vi "Dark Array FGV.vi"(10 "Control":enum16{"get", "add", "reset"}(ring), 11 "Next Dark Measurement In":dbl[][](array[numeric])) -> (3 "All Dark Measurements Out":dbl[][](array[numeric]))   [LabVIEW 2014, in "AvaSpec.lvlib" / "Dark.lvlib"]
doc: "Collects each individual dark measurement and adds to an array to be used to create the dark model"
uses:
  Dark.lvlib
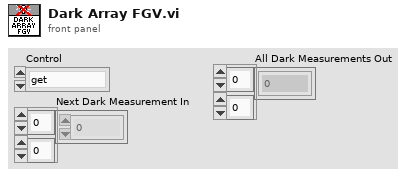
[diagram p1: front panel]
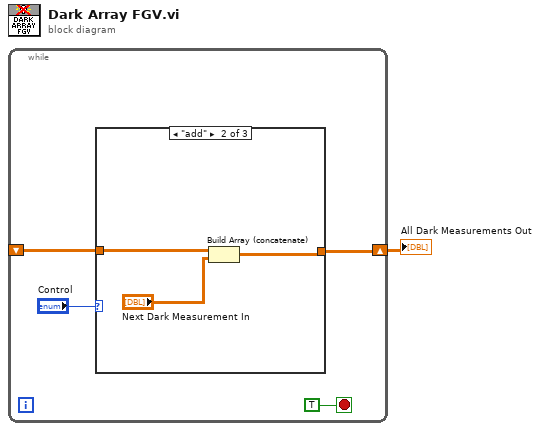
[diagram p0: block diagram]
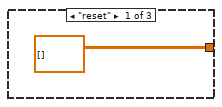
[diagram p2: hidden frame]
diagram:
  n1 = while {
    shift-right: [w3] -> w1
    shift-left: _ -> [w2]
    stop <- TRUE stop-if-true
    n2 = case shown="\"add\"" "Control" {
      tunnel: [dbl[][] [] w7 w10] -> w3
      tunnel: w2 -> [_ w9 w10]
      frame "reset" {
      }
      frame "add" {
        n3 = Build Array (concatenate)(w9, "Next Dark Measurement In") -> (w7:dbl[][])
      }
      frame "get" {
      }
    }
  }
  "All Dark Measurements Out" <- w1
